vi "DriveStraightCommand.vi"(8 "speed":dbl=0.5, 9 "Fwd Bwd":dbl, 10 "Delay ms":u32=500, 11 "distance":dbl) -> ()   [LabVIEW 2014]
uses:
  Robot Global Data.vi
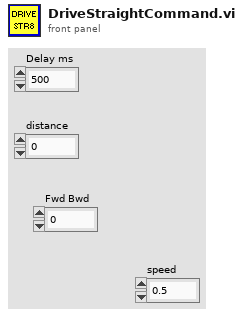
[diagram p1: front panel]
types:
  T1 = typedef "WPI_EncoderDevRef.ctl" = cluster{"DevStatus":errorcluster, "EncoderIndex":T2, "CounterIndex":T3, "DistancePerCount":dbl, "Decoding Type":T4}
  T2 = typedef "FPGA_EncoderIdx.ctl" = enum8{"Enc 0", "Enc 1", "Enc 2", "Enc 3", "Enc 4", "Enc 5", "Enc 6", "Enc 7", "Invalid"}
  T3 = typedef "FPGA_CounterCtrSystemIndex.ctl" = enum8{"Ctr 0", "Ctr 1", "Ctr 2", "Ctr 3", "Ctr 4", "Ctr 5", "Ctr 6", "Ctr 7", "Invalid"}
  T4 = typedef "WPI_EncoderType.ctl" = enum16{"1x", "2x", "4x"}
  T5 = typedef "WPI_GyroDevRef.ctl" = cluster{"DevStatus":errorcluster, "Analog Module":T6, "Analog Channel":T7, "Offset":dbl, "Gain (VoltsPerDegree/Second)":dbl}
  T6 = typedef "FPGA_TypedefAnalogModule.ctl" = enum16{"Controller 1"}
  T7 = typedef "FPGA_AIChannel.ctl" = enum8{"AI 0", "AI 1", "AI 2", "AI 3", "AI MXP 0", "AI MXP 1", "AI MXP 2", "AI MXP 3", "Invalid"}
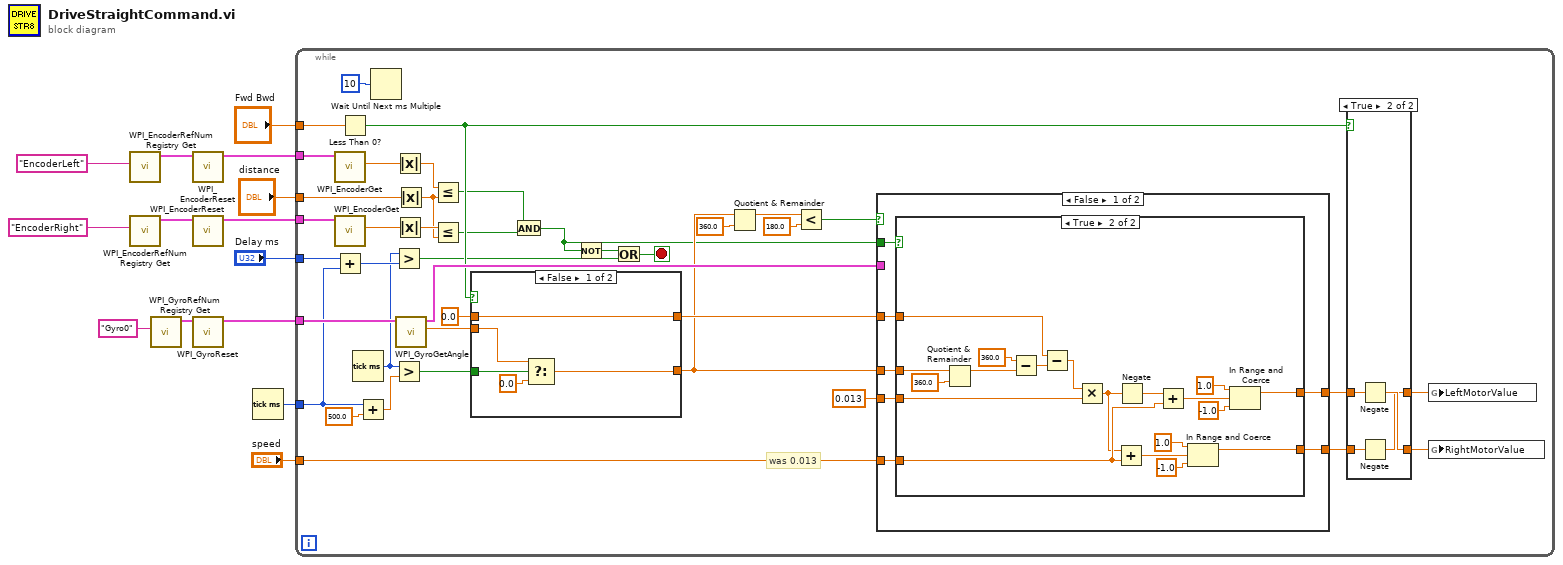
[diagram p0: block diagram]
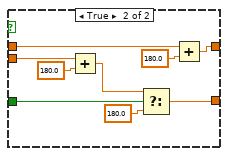
[diagram p3: hidden frame]
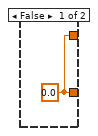
[diagram p4: hidden frame]
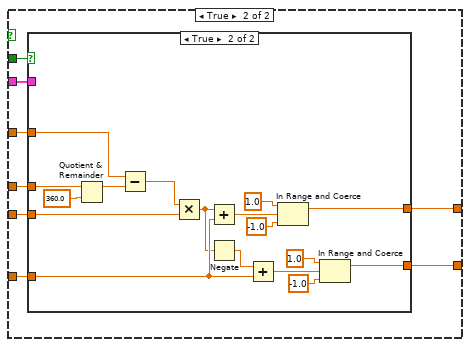
[diagram p5: hidden frame]
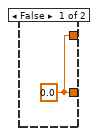
[diagram p6: hidden frame]
diagram:
  n1 = call <vilib>:"WPI_EncoderRefNum Registry Get.vi"("refnum name"="EncoderLeft") -> ("EncoderDevRef"=w13:T1)  [unwired: 9 in, 1 out]
  n2 = call <vilib>:"WPI_EncoderRefNum Registry Get.vi"("refnum name"="EncoderRight") -> ("EncoderDevRef"=w12:T1)  [unwired: 9 in, 1 out]
  n3 = call <vilib>:"WPI_GyroRefNum Registry Get.vi"("refnum name"="Gyro0") -> ("GyroDevRef"=w5:T5)  [unwired: 9 in, 1 out]
  n4 = call <vilib>:"WPI_EncoderReset.vi"("EncoderDevRef"=w13) -> ("EncoderDevRef"=w8:T1)  [unwired: 9 in, 1 out]
  n5 = call <vilib>:"WPI_EncoderReset.vi"("EncoderDevRef"=w12) -> ("EncoderDevRef"=w7:T1)  [unwired: 9 in, 1 out]
  n6 = call <vilib>:"WPI_GyroReset.vi"("GyroDevRef"=w5) -> ("GyroDevRef"=w4:T5)  [unwired: 9 in, 1 out]
  n7 = Tick Count (ms)() -> (millisecond timer value=w2:u32)
  n8 = while {
    tunnel: "speed" -> [w46]
    tunnel: "distance" -> [w35]
    tunnel: w4 -> [w40]
    tunnel: w8 -> [w39]
    tunnel: w7 -> [w38]
    tunnel: "Fwd Bwd" -> [w37]
    tunnel: "Delay ms" -> [w24]
    tunnel: w2 -> [w22]
    stop <- w36 stop-if-true
    # "was 0.013"
    n9 = call <vilib>:"WPI_EncoderGet.vi"("EncoderDevRef"=w39) -> ("Distance"=w47:dbl)  [unwired: 5 in, 5 out]
    n10 = call <vilib>:"WPI_EncoderGet.vi"("EncoderDevRef"=w38) -> ("Distance"=w51:dbl)  [unwired: 5 in, 5 out]
    n11 = Add(x=w24, y=w22) -> (x+y=w26:u32)
    n12 = Less Than 0?(x=w37) -> (x < 0?=w32:bool)
    n13 = Tick Count (ms)() -> (millisecond timer value=w20:u32)
    n14 = Add(x=w22, y=500.0) -> (x+y=w21:dbl)
    n15 = Wait Until Next ms Multiple(millisecond multiple=u32 10 ("milliseconds to wait")) -> ()  [unwired: 1 out]
    n16 = Greater?(x=w20, y=w26) -> (0:w25:bool)
    n17 = Greater?(x=w20, y=w21) -> (0:w19:bool)
    n18 = Absolute Value(x=w47) -> (abs(x)=w52:dbl)
    n19 = Absolute Value(x=w51) -> (abs(x)=w54:dbl)
    n20 = Absolute Value(x=w35) -> (abs(x)=w53:dbl)
    n21 = call <vilib>:"WPI_GyroGetAngle.vi"("GyroDevRef"=w40) -> ("Angle"=w48:dbl, "GyroDevRef"=w44:T5)  [unwired: 7 in, 2 out]
    n22 = Less Or Equal?(x=w52, y=w53) -> (x <= y?=w17:bool)
    n23 = Less Or Equal?(x=w54, y=w53) -> (x <= y?=w16:bool)
    n24 = case shown="False" w32 {
      tunnel: w48 -> [w64 w74]
      tunnel: [w63 w68] -> w34
      tunnel: 0.0 ("wanted angle") -> [w65 w70]
      tunnel: [w65 w72] -> w50
      tunnel: w19 -> [w62 w67]
      frame False {
        n25 = Select(t=w64, s=w62, f=0.0) -> (s? t:f=w63:dbl)
      }
      frame True {
        n26 = Add(x=w74, y=180.0) -> (x+y=w69:dbl)
        n27 = Select(t=w69, s=w67, f=180.0) -> (s? t:f=w68:dbl)
        n28 = Add(x=w70, y=180.0) -> (x+y=w72:dbl)
      }
    }
    n29 = And(x=w17, y=w16) -> (x .and. y?=w18:bool)
    n30 = Not(x=w18) -> (.not. x?=w15:bool)
    n31 = Or(x=w15, y=w25) -> (x .or. y?=w36:bool)
    n32 = Quotient & Remainder(x=w34, y=360.0) -> (x-y*floor(x/y)=w41:dbl)  [unwired: 1 out]
    n33 = Less?(x=w41, y=180.0) -> (x < y?=w31:bool)
    n34 = case shown="False" w31 {
      tunnel: w50 -> [w80 w109]
      tunnel: [w76 w103] -> w28
      tunnel: w46 -> [w81 w108]
      tunnel: 0.013 ("Kp Gain") -> [w78 w107]
      tunnel: w18 -> [w77 w106]
      tunnel: [w75 w102] -> w27
      tunnel: w44 -> [_ w105]
      tunnel: w34 -> [w79 w104]
      frame False {
        n35 = case shown="True" w77 {
          tunnel: w81 -> [_ w89]
          tunnel: w80 -> [_ w94]
          tunnel: w79 -> [_ w93]
          tunnel: w78 -> [_ w88]
          tunnel: [w82 w84] -> w75
          tunnel: [w82 w83] -> w76
          frame False {
            w82 = 0.0
          }
          frame True {
            n36 = Quotient & Remainder(x=w93, y=360.0) -> (x-y*floor(x/y)=w91:dbl)  [unwired: 1 out]
            n37 = Subtract(x=360.0, y=w91) -> (x-y=w90:dbl)
            n38 = Subtract(x=w94, y=w90) -> (x-y=w85:dbl)
            n39 = Multiply(x=w85, y=w88) -> (x*y=w86:dbl)
            n40 = Add(x=w86, y=w89) -> (x+y=w98:dbl)
            n41 = Negate(x=w86) -> (-x=w87:dbl)
            n42 = Add(x=w87, y=w89) -> (x+y=w95:dbl)
            n43 = In Range and Coerce(upper limit=1.0, x=w98, lower limit=-1.0) -> (coerced(x)=w84:dbl)  [unwired: 1 out]
            n44 = In Range and Coerce(upper limit=1.0, x=w95, lower limit=-1.0) -> (coerced(x)=w83:dbl)  [unwired: 1 out]
          }
        }
      }
      frame True {
        n45 = case shown="True" w106 {
          tunnel: w105 -> [_ _]
          tunnel: w109 -> [_ w124]
          tunnel: [w110 w112] -> w103
          tunnel: w108 -> [_ w117]
          tunnel: w107 -> [_ w121]
          tunnel: [w110 w111] -> w102
          tunnel: w104 -> [_ w118]
          frame False {
            w110 = 0.0 ("output")
          }
          frame True {
            n46 = Quotient & Remainder(x=w118, y=360.0) -> (x-y*floor(x/y)=w125:dbl)  [unwired: 1 out]
            n47 = Subtract(x=w124, y=w125) -> (x-y=w113:dbl)
            n48 = Multiply(x=w113, y=w121) -> (x*y=w116:dbl)
            n49 = Add(x=w116, y=w117) -> (x+y=w122:dbl)
            n50 = Negate(x=w116) -> (-x=w114:dbl)
            n51 = Add(x=w114, y=w117) -> (x+y=w115:dbl)
            n52 = In Range and Coerce(upper limit=1.0, x=w122, lower limit=-1.0) -> (coerced(x)=w112:dbl)  [unwired: 1 out]
            n53 = In Range and Coerce(upper limit=1.0, x=w115, lower limit=-1.0) -> (coerced(x)=w111:dbl)  [unwired: 1 out]
          }
        }
      }
    }
    n54 = case shown="True" w32 {
      tunnel: [w56 w57] -> w30
      tunnel: [w55 w58] -> w29
      tunnel: w28 -> [w56 w60]
      tunnel: w27 -> [w55 w59]
      frame False {
      }
      frame True {
        n55 = Negate(x=w60) -> (-x=w58:dbl)
        n56 = Negate(x=w59) -> (-x=w57:dbl)
      }
    }
    n57 = global write "Robot Global Data.vi" "LeftMotorValue"(w30) -> ()
    n58 = global write "Robot Global Data.vi" "RightMotorValue"(w29) -> ()
  }
